vi "BinF_SaveData.vi"(6 "Channel number":i64, 7 "BinF File Settings":T1={"Data Representation"=enum."I16", "# columns (samples per channel)"=300, "# rows (channels)"=150, "# pre-trigger samples"=20, "Sample rate"=1000.0, "ADC offset"=256, "Scale factor"=0.001}, 8 "error in":errorcluster, 9 "Channel Data":i16[](array[numeric]), 10 "Start":i64, 11 "refnum":refnum<file>) -> (0 "error out":errorcluster, 3 "refnum out":refnum<file>)   [LabVIEW 2015]
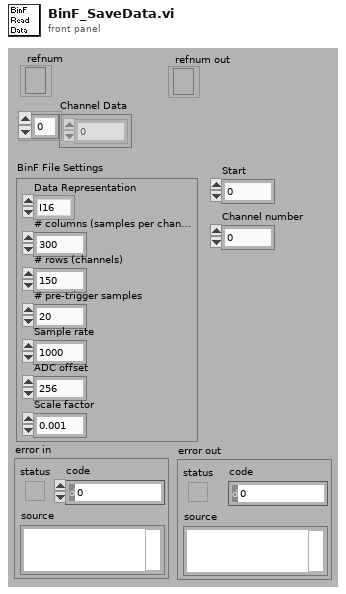
[diagram p1: front panel]
types:
  T1 = cluster{"Data Representation":enum16{"Undefined", "I8", "I16", "I32", "I64", "U8", "U16", "U32", "U64", "SGL", "DBL", "EXT"}, "# columns (samples per channel)":i64, "# rows (channels)":i64, "# pre-trigger samples":i64, "Sample rate":dbl, "ADC offset":i32, "Scale factor":dbl}
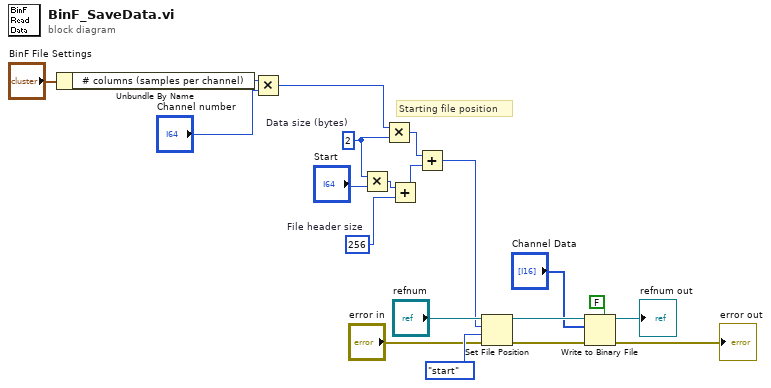
[diagram p0: block diagram]
diagram:
  w15 = i64 256  # File header size
  w6 = i64 2  # Data size (bytes)
  # "Starting file position"
  n1 = Unbundle By Name("BinF File Settings") -> ("# columns (samples per channel)"=w10:i64)
  n2 = Multiply(x=w10, y="Channel number") -> (x*y=w5:i64)
  n3 = Multiply(x=w6, y="Start") -> (x*y=w16:i64)
  n4 = Multiply(x=w5, y=w6) -> (x*y=w12:i64)
  n5 = Add(x=w16, y=w15) -> (x+y=w13:i64)
  n6 = Add(x=w12, y=w13) -> (x+y=w11:i64)
  n7 = Set File Position(offset (in bytes) (0)=w11, refnum="refnum", from (0:start)=enum16{"start", "end", "current"}."start", error in="error in") -> (refnum out=w3:refnum<file>, error out=w17:errorcluster)
  n8 = Write to Binary File(file (use dialog)=w3, data="Channel Data", error in=w17, 5:FALSE ("prepend array or string size? (T)")) -> (refnum out=→"refnum out":refnum<file>, error out=→"error out":errorcluster)  [unwired: 2 in, 1 out]
